vi "CheckonIdle.vi"(5 "MessageQueue(MA)":refnum<queue>, 7 "MessageQueue(Class)":refnum<queue>, 8 "error in (no error)":errorcluster, 9 "Timeout (10s)":dbl=10.0 min=0.0 max=10.0, 10 "ChangeOccured? (F)":bool, 11 "AcPwrBase in":refnum<class "AcPwrBase.lvclass">) -> (0 "Error Out":errorcluster, 2 "Write?":bool, 3 "AcPwrBase out":refnum<class "AcPwrBase.lvclass">)   [LabVIEW 2018, in "AcPwrPlugins.lvlib"]
doc: "This VI ensures the acquisition loop is in the idle state before reconfiguring the instrument. Some instruments will error and lock up if a user tries to reconfigure the instrument while the instrument is in acquisition mode."
uses:
  AcPwrPlugins.lvlib
  AcPwrBaseClass/AcPwrBase.lvclass
  clMessage.ctl
  CheckOnIdleEnum.ctl
  EnqueueEnum.ctl
  <vilib>/Utility/error.llb/Error Cluster From Error Code.vi
  <vilib>/ErrorRing/Error Ring.xnode
panel:
  out "InRun?":bool=TRUE
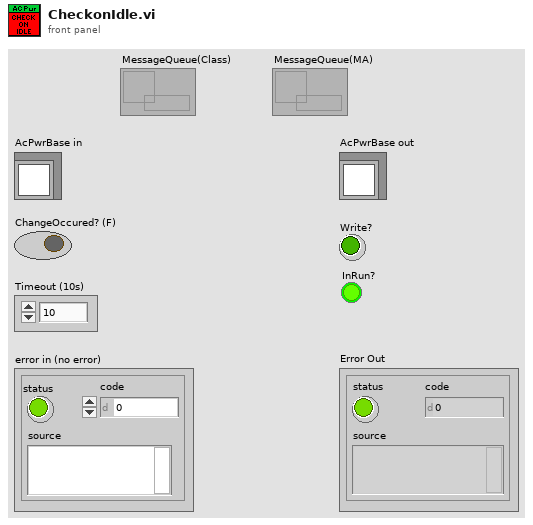
[diagram p1: front panel]
types:
  T1 = typedef "AcPwrPlugins.lvlib/CheckOnIdleEnum.ctl" = enum16{"CheckOnState", "WriteToClassAndExit", "InIdle", "SetToStop", "Error", "SetToStart", "Exit"}
  T2 = typedef "AcPwrPlugins.lvlib/EnqueueEnum.ctl" = enum16{"LossyEnqueue", "EnqueueAtFront", "Enqueue"}
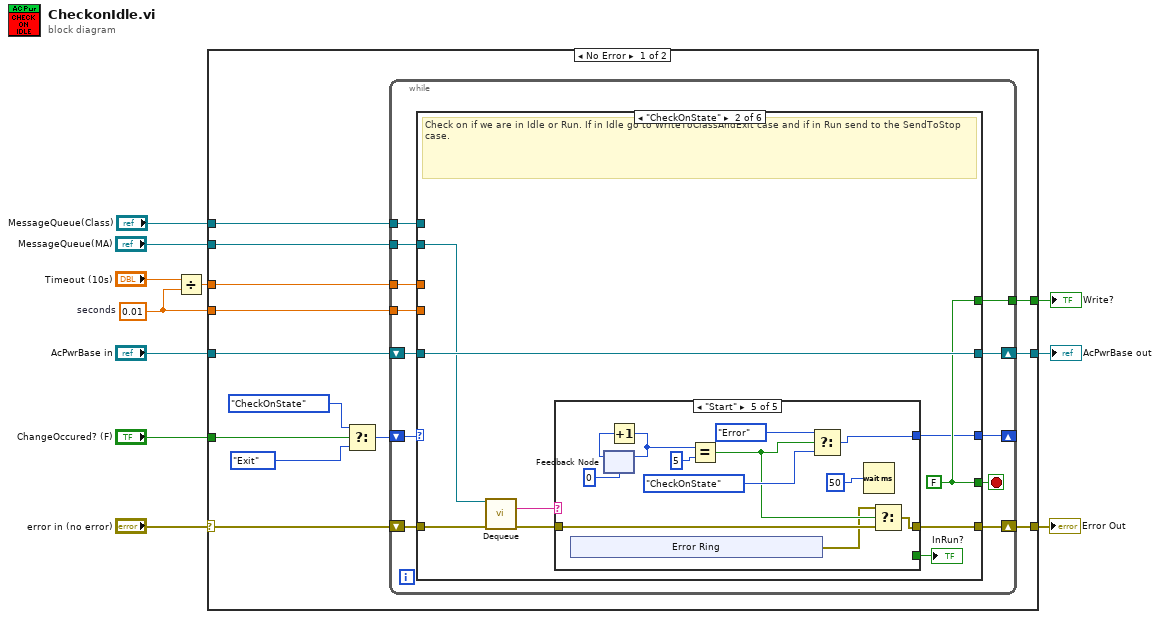
[diagram p0: block diagram]
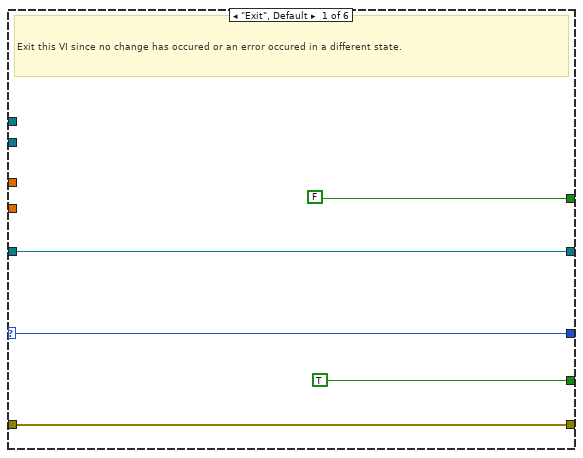
[diagram p2: hidden frame]
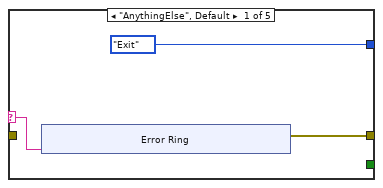
[diagram p3: hidden frame]
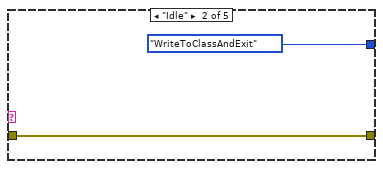
[diagram p4: hidden frame]
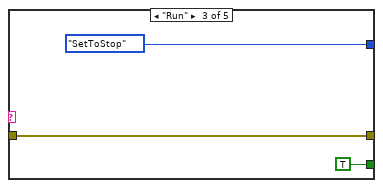
[diagram p5: hidden frame]
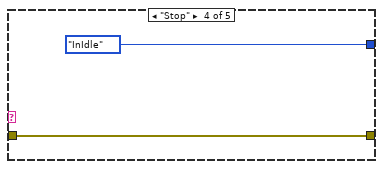
[diagram p6: hidden frame]
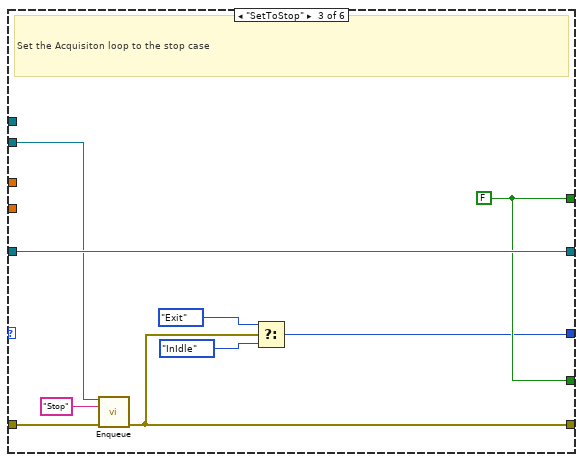
[diagram p7: hidden frame]
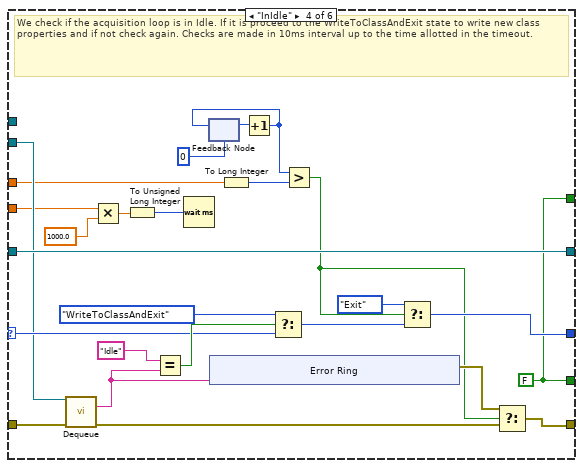
[diagram p8: hidden frame]
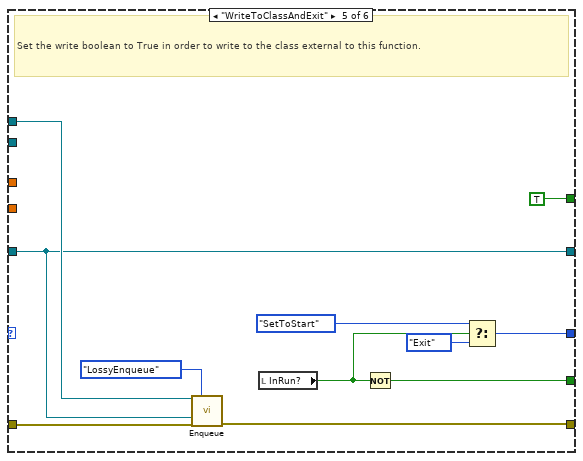
[diagram p9: hidden frame]
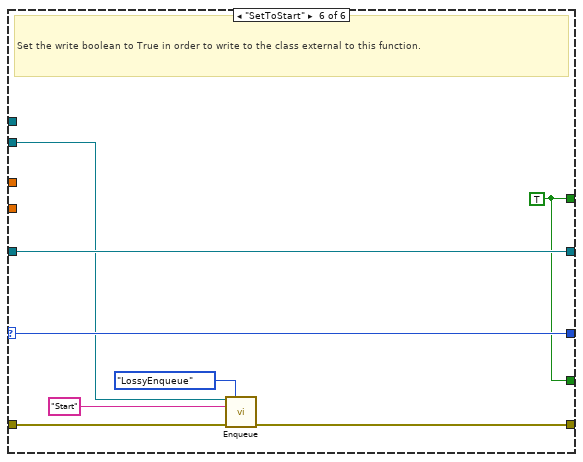
[diagram p10: hidden frame]
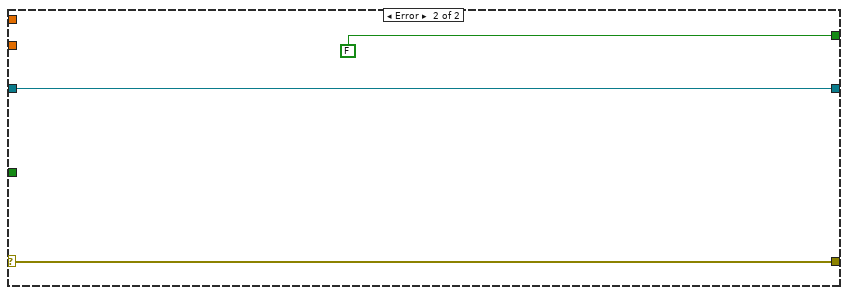
[diagram p11: hidden frame]
diagram:
  w2 = 0.01  # seconds
  n1 = Divide(x="Timeout (10s)", y=w2) -> (x/y=w7:dbl)
  n2 = case shown="No Error" "error in (no error)" {
    selector: "error in (no error)" -> [w23 w147]
    tunnel: "ChangeOccured? (F)" -> [w22 _]
    tunnel: "AcPwrBase in" -> [w21 w146]
    tunnel: [w20 w147] -> w11
    tunnel: w7 -> [w19 _]
    tunnel: [w18 w146] -> w4
    tunnel: [w17 FALSE ("Set? (f)")] -> w6
    tunnel: "MessageQueue(MA)" -> [w16 _]
    tunnel: w2 -> [w15 _]
    tunnel: "MessageQueue(Class)" -> [w12 _]
    frame No Error {
      n3 = Select(t=CheckOnIdleEnum."CheckOnState" ("Enum"), s=w22, f=CheckOnIdleEnum."Exit" ("Enum")) -> (s? t:f=w24:T1)
      n4 = while {
        shift-right: [w31] -> _
        shift-left: w24 -> [w36]
        shift-right: [w33] -> w18
        shift-left: w21 -> [w34]
        shift-right: [w32] -> w20
        shift-left: w23 -> [w35]
        tunnel: w19 -> [w29]
        tunnel: [w28] -> w17
        tunnel: w16 -> [w27]
        tunnel: w15 -> [w26]
        tunnel: w12 -> [w25]
        stop <- w30 stop-if-true
        n5 = case shown="\"CheckOnState\"" w36 {
          selector: w36 -> [w40 _ _ w117 _ w144]
          tunnel: w35 -> [w41 w45 w91 w97 w130 w143]
          tunnel: w34 -> [w39 w50 w93 w116 w126 w141]
          tunnel: [w41 w46 w88 w102 w129 w142] -> w32
          tunnel: [w39 w50 w93 w116 w126 w141] -> w33
          tunnel: [w40 w47 w87 w111 w135 w144] -> w31
          tunnel: [TRUE w48 w92 w104 w134 w140] -> w30
          tunnel: w29 -> [_ _ _ w98 _ _]
          tunnel: [FALSE ("Set? (f)") w48 w92 w104 TRUE ("Set? (f)") w140] -> w28
          tunnel: w27 -> [_ w49 w90 w110 _ w139]
          tunnel: w26 -> [_ _ _ w107 _ _]
          tunnel: w25 -> [_ _ _ _ w127 _]
          frame "Exit", Default {
            # "Exit this VI since no change has occured or an error occured in a different state."
          }
          frame "CheckOnState" {
            w48 = FALSE
            # "Check on if we are in Idle or Run. If in Idle go to WriteToClassAndExit case and if in Run send to the SendToStop case."
            n6 = call "Dequeue.vi"("MessageQueue"=w49, "error in (no error)"=w45) -> ("Message"=w44:string, "error out"=w43:errorcluster)  [unwired: 9 in, 3 out]
            n7 = case shown="\"Start\"" w44 {
              selector: w44 -> [w51 _ _ _ _]
              tunnel: [CheckOnIdleEnum."Exit" ("Enum") CheckOnIdleEnum."WriteToClassAndExit" ("Enum") CheckOnIdleEnum."SetToStop" ("Enum") CheckOnIdleEnum."InIdle" ("Enum") w75] -> w47
              tunnel: w43 -> [_ w61 w64 w66 w74]
              tunnel: [w52 w61 w64 w66 w73] -> w46
              tunnel: [_ _ TRUE _ _] -> w42
              frame "AnythingElse", Default {
                n8 = xnode "Error Ring"("parameter 0"=w51) -> ("error out"=w52:errorcluster)
              }
              frame "Idle" {
              }
              frame "Run" {
              }
              frame "Stop" {
              }
              frame "Start" {
                n9 = xnode "Error Ring"() -> ("error out"=w69:errorcluster)
                n10 = feedback #1(0) -> (w78:i32)
                n11 = Increment(x=w78) -> (x+1=w72:i32)
                n12 = feedback-in #1(w72) -> ()
                n13 = Equal?(x=w72, y=5 ("x")) -> (x = y?=w70:bool)
                n14 = Select(t=CheckOnIdleEnum."Error" ("Enum"), s=w70, f=CheckOnIdleEnum."CheckOnState" ("Enum")) -> (s? t:f=w75:T1)
                n15 = Wait (ms)(milliseconds to wait=u32 50) -> ()  [unwired: 1 out]
                n16 = Select(t=w69, s=w70, f=w74) -> (s? t:f=w73:errorcluster)
              }
            }
            "InRun?" <- w42
          }
          frame "SetToStop" {
            w92 = FALSE
            # "Set the Acquisiton loop to the stop case"
            n17 = call "Enqueue.vi"("MessageQueue"=w90, "Message"="Stop", "error in (no error)"=w91) -> ("error out"=w88:errorcluster)  [unwired: 11 in, 1 out]
            n18 = Select(t=CheckOnIdleEnum."Exit" ("Enum"), s=w88, f=CheckOnIdleEnum."InIdle" ("Enum")) -> (s? t:f=w87:T1)
          }
          frame "InIdle" {
            w104 = FALSE
            # "We check if the acquisition loop is in Idle. If it is proceed to the WriteToClassAndExit state to write new class properties and if not check again. Checks are made in 10ms interval up to the time allotted in the timeout."
            n19 = call "Dequeue.vi"("MessageQueue"=w110, "error in (no error)"=w97) -> ("Message"=w95:string, "error out"=w96:errorcluster)  [unwired: 9 in, 3 out]
            n20 = Multiply(x=w107, y=1000.0) -> (x*y=w106:dbl)
            n21 = To Unsigned Long Integer(number=w106) -> (unsigned 32bit integer=w109:u32)
            n22 = Equal?(x="Idle" ("State In"), y=w95) -> (x = y?=w118:bool)
            n23 = Wait (ms)(milliseconds to wait=w109) -> ()  [unwired: 1 out]
            n24 = feedback #2(0) -> (w114:i32)
            n25 = xnode "Error Ring"("parameter 0"=w95) -> ("error out"=w103:errorcluster)
            n26 = To Long Integer(number=w98) -> (32bit integer=w99:i32)
            n27 = Increment(x=w114) -> (x+1=w113:i32)
            n28 = feedback-in #2(w113) -> ()
            n29 = Select(t=CheckOnIdleEnum."WriteToClassAndExit" ("Enum"), s=w118, f=w117) -> (s? t:f=w112:T1)
            n30 = Greater?(x=w113, y=w99) -> (0:w101:bool)
            n31 = Select(t=CheckOnIdleEnum."Exit" ("Enum"), s=w101, f=w112) -> (s? t:f=w111:T1)
            n32 = Select(t=w103, s=w101, f=w96) -> (s? t:f=w102:errorcluster)
          }
          frame "WriteToClassAndExit" {
            # "Set the write boolean to True in order to write to the class external to this function."
            n33 = call "Enqueue.vi"("MessageQueue"=w127, "EnqueueType (Enqueue)"=EnqueueEnum."LossyEnqueue", "AcPwrBase"=w126, "error in (no error)"=w130) -> ("error out"=w129:errorcluster)  [unwired: 10 in, 1 out]
            n34 = local read "InRun?"() -> (w133:bool)
            n35 = Not(x=w133) -> (.not. x?=w134:bool)
            n36 = Select(t=CheckOnIdleEnum."SetToStart" ("Enum"), s=w133, f=CheckOnIdleEnum."Exit") -> (s? t:f=w135:T1)
          }
          frame "SetToStart" {
            w140 = TRUE ("Set? (f)")
            # "Set the write boolean to True in order to write to the class external to this function."
            n37 = call "Enqueue.vi"("MessageQueue"=w139, "EnqueueType (Enqueue)"=EnqueueEnum."LossyEnqueue", "Message"="Start", "error in (no error)"=w143) -> ("error out"=w142:errorcluster)  [unwired: 10 in, 1 out]
          }
        }
      }
    }
    frame Error {
    }
  }
  "Error Out" <- w11
  "Write?" <- w6
  "AcPwrBase out" <- w4
